vi "time.vi"(10 "x":u16) -> (2 "Time":string="00:00")   [LabVIEW 2019]
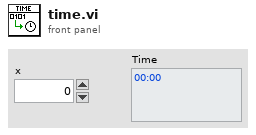
[diagram p1: front panel]
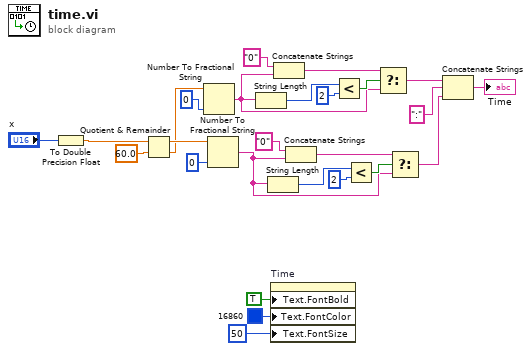
[diagram p0: block diagram]
diagram:
  n1 = To Double Precision Float(number="x") -> (double precision float=w1:dbl)
  n2 = Quotient & Remainder(x=w1, y=60.0) -> (x-y*floor(x/y)=w13:dbl, floor(x/y)=w12:dbl)
  n3 = Number To Fractional String(number=w12, precision (6)=i16 0) -> (F-format string=w16:string)  [unwired: 2 in]
  n4 = Number To Fractional String(number=w13, precision (6)=i16 0) -> (F-format string=w5:string)  [unwired: 2 in]
  n5 = String Length(string=w16) -> (length=w21:i32)
  n6 = String Length(string=w5) -> (length=w7:i32)
  n7 = property on="Time" class="Str"("Text.FontBold"=TRUE ("Text.Font:Bold"), "Text.FontColor"=u32 16860 ("Text.Font:Color"), "Text.FontSize"=u32 50 ("Text.Font:Size")) -> ()  [unwired: 2 in, 2 out]
  n8 = Concatenate Strings("0" ("string"), w16) -> (w18:string)
  n9 = Concatenate Strings("0" ("string"), w5) -> (w10:string)
  n10 = Less?(x=w21, y=2) -> (x < y?=w19:bool)
  n11 = Less?(x=w7, y=2) -> (x < y?=w9:bool)
  n12 = Select(t=w18, s=w19, f=w16) -> (s? t:f=w15:string)
  n13 = Select(t=w10, s=w9, f=w5) -> (s? t:f=w6:string)
  n14 = Concatenate Strings(w15, ":" ("string"), w6) -> (→"Time":string)
